vi "7.4.1.vi"() -> ()   [LabVIEW 2018]
panel:
  in  "경로":path
  out "랜덤 데이터":dbl[](graph)
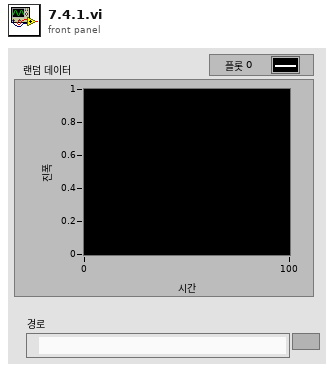
[diagram p1: front panel]
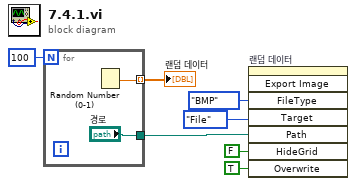
[diagram p0: block diagram]
diagram:
  n1 = for {
    N: 100 -> [_]
    tunnel: [w9] -> w6 mode=indexing
    tunnel: ["경로"] -> w3
    n2 = Random Number (0-1)() -> (number: 0 to 1=w9:dbl)
  }
  "랜덤 데이터" <- w6
  n3 = invoke on="랜덤 데이터" class="WFChart (엄격한)" method="Export Image"("FileType"=enum32{"BMP", "EPS", "EMF", "PICT"}."BMP" ("파일 타입"), "Target"=enum32{"File", "Clipboard"}."File" ("타겟"), "Path"=w3, "HideGrid"=FALSE ("눈금 숨기기"), "Overwrite"=TRUE ("항상 덮어쓰기")) -> ()  [unwired: 3 in, 8 out]
